vi "Joystick Angle-Mag.vi"(10 "Yaxis":i16, 11 "Xaxis":i16) -> (2 "Mag":i16, 3 "Angle":dbl)   [LabVIEW 2013, in "ProcessorHelperFunctions.lvlib"]
uses:
  ProcessorHelperFunctions.lvlib
  <vilib>/express/express arith-compare/Formula/XNode/ExpressFormulaBlockNode.xnode
  <vilib>/ptbypt/NI_PtbyPt.lvlib
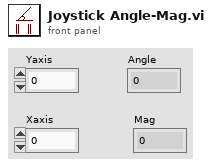
[diagram p1: front panel]
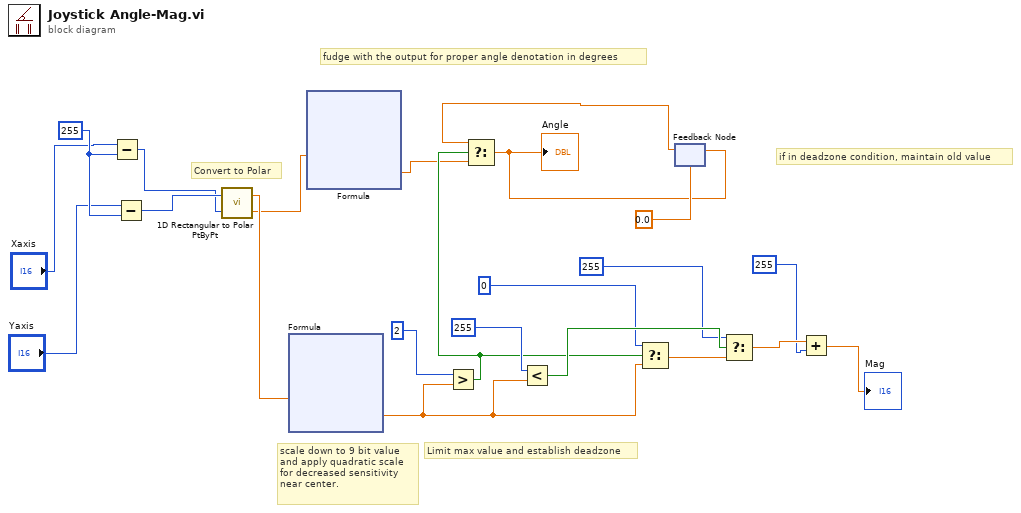
[diagram p0: block diagram]
diagram:
  w7 = 255
  # "if in deadzone condition, maintain old value"
  # "fudge with the output for proper angle denotation in degrees"
  # "scale down to 9 bit value\nand apply quadratic scale \nfor decreased sensitivity\nnear center."
  # "Limit max value and establish deadzone"
  # "Convert to Polar"
  n1 = Subtract(x="Xaxis", y=w7) -> (x-y=w3:i32)
  n2 = Subtract(x="Yaxis", y=w7) -> (x-y=w4:i32)
  n3 = call <vilib>:"1D Rectangular to Polar PtByPt.vi"("y"=w3, "x"=w4) -> ("phase"=w21:dbl, "magnitude"=w22:dbl)
  n4 = xnode "Formula"("Input"=w22) -> ("Result"=w13:dbl)  [unwired: 1 in, 1 out]
  n5 = xnode "Formula"("RadAng"=w21) -> ("Result"=w10:dbl)  [unwired: 1 in, 1 out]
  n6 = Greater?(x=2, y=w13) -> (0:w12:bool)
  n7 = Less?(x=255, y=w13) -> (x < y?=w18:bool)
  n8 = Select(t=0, s=w12, f=w13) -> (s? t:f=w20:dbl)
  n9 = feedback #1(0.0) -> (w11:dbl)
  n10 = Select(t=w11, s=w12, f=w10) -> (s? t:f=w8:dbl)
  "Angle" <- w8
  n11 = feedback-in #1(w8) -> ()
  n12 = Select(t=255, s=w18, f=w20) -> (s? t:f=w19:dbl)
  n13 = Add(x=w19, y=255) -> (x+y=→"Mag":dbl)
